vi "FV_motor_set.vi"(6 "delay  (sec)":dbl=0.01 caption="Delay Time (s)", 8 "error in":errorcluster, 10 "command":string="FP", 11 "VISA in":refnum<visa-resource-name>) -> (0 "error out":errorcluster, 3 "VISA out":refnum<visa-resource-name>)   [LabVIEW 2019]
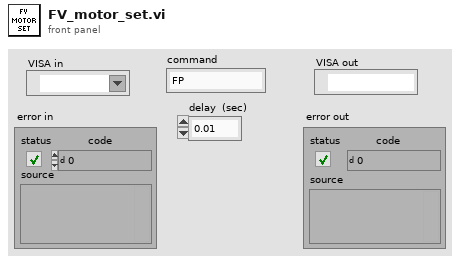
[diagram p1: front panel]
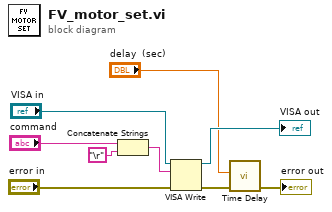
[diagram p0: block diagram]
diagram:
  n1 = Concatenate Strings("command", "\r") -> (w9:string)
  n2 = VISA Write(VISA resource name="VISA in", write buffer=w9, error in (no error)="error in") -> (VISA resource name out=→"VISA out":refnum<visa-resource-name>, error out=w5:errorcluster)  [unwired: 1 out]
  n3 = call "Time Delay"("error in (no error)"=w5, "Delay Time (s)"="delay  (sec)") -> ("error out"=→"error out":errorcluster)  [unwired: 9 in]
